vi "SplineHelp_GetCubicCtrlVectorsFromWayPts.vi"(9 "Enging POSE":T2={"TRANSLATION"={"X"=0.0, "Y"=0.0}, "ROTATION"={"VALUE"=0.0, "COS"=1.0, "SIN"=0.0}} {"ROTATION"."SIN" format="%13.4f"; "ROTATION"."COS" format="%13.4f"; "ROTATION"."VALUE" format="%13.4f"; "TRANSLATION"."Y" format="%14.3f"; "TRANSLATION"."X" format="%14.3f"}, 10 "Interior WAYPOINTS":T3[](array[typedef]) {"Y" format="%14.3f"; "X" format="%14.3f"}, 11 "Starting POSE":T2={"TRANSLATION"={"X"=0.0, "Y"=0.0}, "ROTATION"={"VALUE"=0.0, "COS"=1.0, "SIN"=0.0}} {"ROTATION"."SIN" format="%13.4f"; "ROTATION"."COS" format="%13.4f"; "ROTATION"."VALUE" format="%13.4f"; "TRANSLATION"."Y" format="%14.3f"; "TRANSLATION"."X" format="%14.3f"}) -> (3 "SplineControlVectors":T1[](array[typedef]))   [LabVIEW 2019, in "Trajectory_Library.lvlib"]
doc: "Returns 2 cubic control vectors from a set of exterior waypoints and interior translations.\n\nParameters: \n - startPose - The starting pose.\n - interiorWaypoints - The interior waypoints.\n - endPose - The ending pose.\n\nReturns:\n - SplineControlVectors - Array of cubic control vectors."
uses:
  Trajectory_Library.lvlib
  TypeDef/POSE2D.ctl
  TypeDef/TRANSLATION2D.ctl
  TypeDef/ROTATION2D.ctl
  TypeDef/SPLINE_CTRL_VECTOR.ctl
  Util_CalcDist.vi
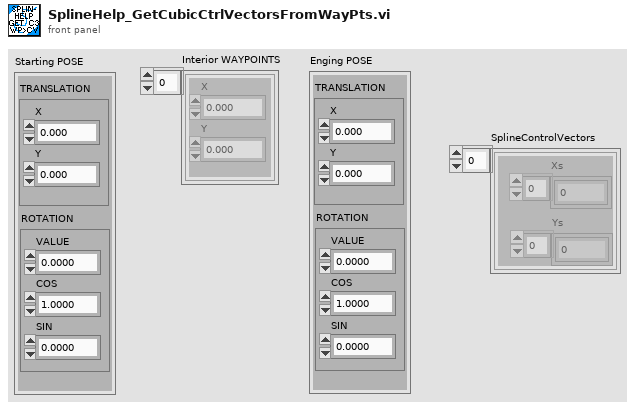
[diagram p1: front panel]
types:
  T1 = typedef "Trajectory_Library.lvlib/SPLINE_CTRL_VECTOR.ctl" = cluster{"Xs":dbl[], "Ys":dbl[]}
  T2 = typedef "Trajectory_Library.lvlib/POSE2D.ctl" = cluster{"TRANSLATION":T3, "ROTATION":T4}
  T3 = typedef "Trajectory_Library.lvlib/TRANSLATION2D.ctl" = cluster{"X":dbl, "Y":dbl}
  T4 = typedef "Trajectory_Library.lvlib/ROTATION2D.ctl" = cluster{"VALUE":dbl, "COS":dbl, "SIN":dbl}
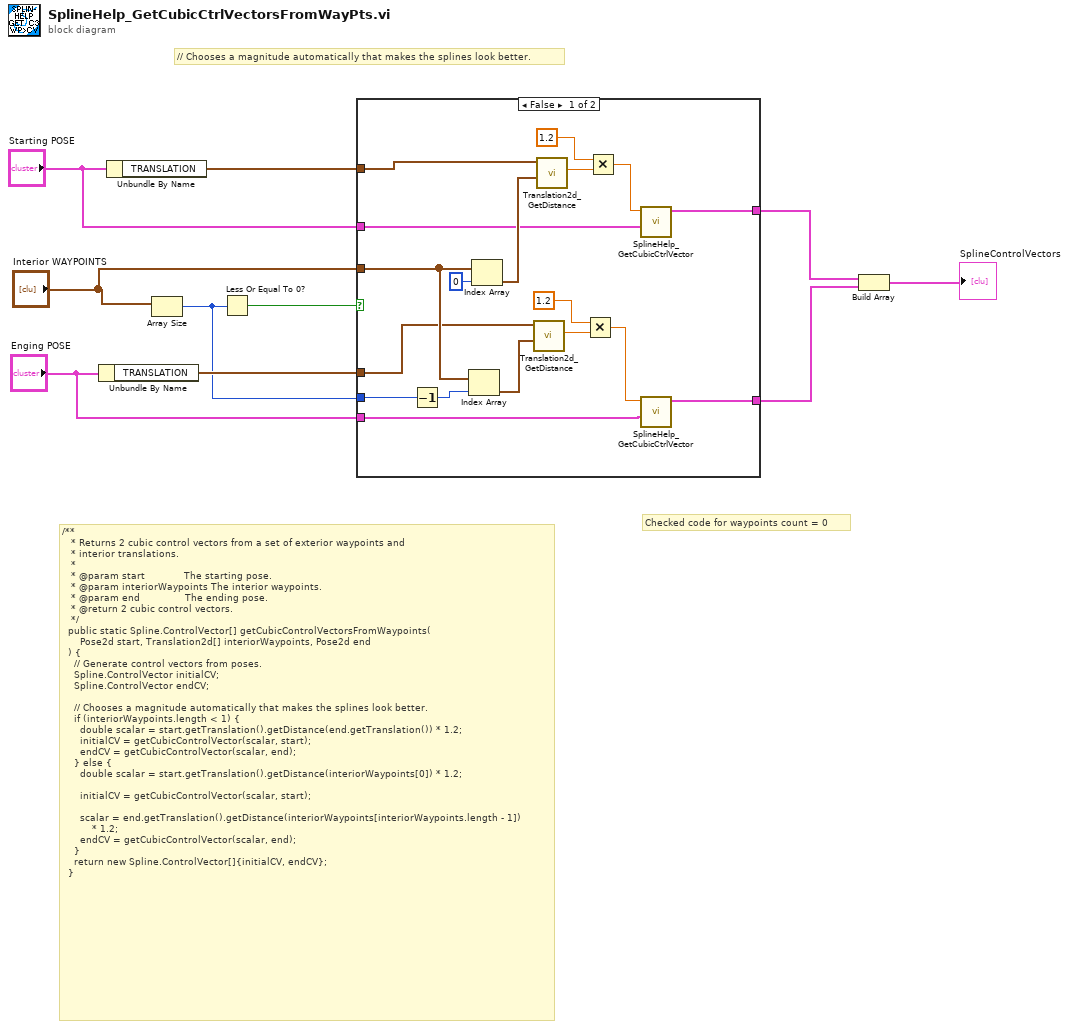
[diagram p0: block diagram]
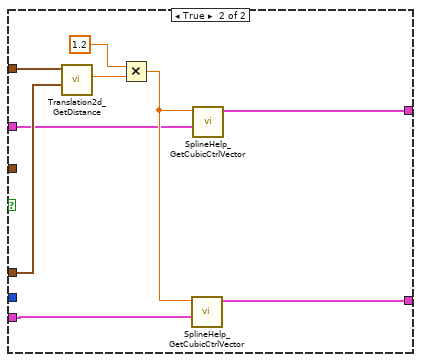
[diagram p2: hidden frame]
diagram:
  # "Checked code for waypoints count = 0"
  # "// Chooses a magnitude automatically that makes the splines look better."
  # "/**\n   * Returns 2 cubic control vectors from a set of exterior waypoints and\n   * interior translations.\n   *\n   * @param start             The starting pose.\n   * @param interiorWaypoints The interior waypoints.\n   * @param end               The ending pose.\n   * @return 2 cubic control vectors.\n   */\n  public static Spline.ControlVector[] getCubicControlVectorsFromWaypoints(\n      Pose2d start, Translation2d[] interiorWaypoints, Pose2d end\n  ) {\n    // Generate control vectors from poses.\n    Spline.ControlVector initialCV;\n    Spline.ControlVector endCV;\n\n    // Chooses a magnitude automatically that makes the splines look better.\n    if (interiorWaypoints.length < 1) {\n      double scalar = start.getTranslation().getDistance(end.getTranslation()) * 1.2;\n      initialCV = getCubicControlVector(scalar, start);\n      endCV = getCubicControlVector(scalar, end);\n    } else {\n      double scalar = start.getTranslation().getDistance(interiorWaypoints[0]) * 1.2;\n\n      initialCV = getCubicControlVector(scalar, start);\n\n      scalar = end.getTranslation().getDistance(interiorWaypoints[interiorWaypoints.length - 1])\n          * 1.2;\n      endCV = getCubicControlVector(scalar, end);\n    }\n    return new Spline.ControlVector[]{initialCV, endCV};\n  }"
  n1 = Unbundle By Name("Enging POSE") -> ("TRANSLATION"=w9:T3)
  n2 = Unbundle By Name("Starting POSE") -> ("TRANSLATION"=w8:T3)
  n3 = Array Size(array="Interior WAYPOINTS") -> (size(s)=w4:i32)
  n4 = Less Or Equal To 0?(x=w4) -> (x <= 0?=w10:bool)
  n5 = case shown="False" w10 {
    tunnel: w9 -> [w13 w36]
    tunnel: w8 -> [w24 w37]
    tunnel: "Starting POSE" -> [w17 w31]
    tunnel: "Enging POSE" -> [w16 w32]
    tunnel: [w19 w30] -> w3
    tunnel: [w20 w29] -> w2
    tunnel: "Interior WAYPOINTS" -> [w23 _]
    tunnel: w4 -> [w12 _]
    frame False {
      n6 = Decrement(x=w12) -> (x-1=w15:i32)
      n7 = Index Array(array=w23, index=w15) -> (element=w14:T3)
      n8 = Index Array(array=w23, index=0) -> (element=w25:T3)
      n9 = call "Translation2d_GetDistance.vi"("other Translation"=w14, "In Translation"=w13) -> ("Distance"=w22:dbl)  [unwired: 9 in]
      n10 = call "Translation2d_GetDistance.vi"("other Translation"=w25, "In Translation"=w24) -> ("Distance"=w28:dbl)  [unwired: 9 in]
      n11 = Multiply(x=1.2, y=w22) -> (x*y=w11:dbl)
      n12 = Multiply(x=1.2, y=w28) -> (x*y=w18:dbl)
      n13 = call "SplineHelp_GetCubicCtrlVector.vi"("Input POSE"=w17, "Scalar"=w18) -> ("resultSpline_Ctrl_Vector"=w19:T1)  [unwired: 9 in]
      n14 = call "SplineHelp_GetCubicCtrlVector.vi"("Input POSE"=w16, "Scalar"=w11) -> ("resultSpline_Ctrl_Vector"=w20:T1)  [unwired: 9 in]
    }
    frame True {
      n15 = call "Translation2d_GetDistance.vi"("other Translation"=w36, "In Translation"=w37) -> ("Distance"=w35:dbl)  [unwired: 9 in]
      n16 = Multiply(x=1.2, y=w35) -> (x*y=w33:dbl)
      n17 = call "SplineHelp_GetCubicCtrlVector.vi"("Input POSE"=w32, "Scalar"=w33) -> ("resultSpline_Ctrl_Vector"=w29:T1)  [unwired: 9 in]
      n18 = call "SplineHelp_GetCubicCtrlVector.vi"("Input POSE"=w31, "Scalar"=w33) -> ("resultSpline_Ctrl_Vector"=w30:T1)  [unwired: 9 in]
    }
  }
  n19 = Build Array(w3, w2) -> (→"SplineControlVectors":T1[])
